vi "Sub_kalman_discrete_model.vi"() -> ()   [LabVIEW 2021]
uses:
  <vilib>/Analysis/Matrix/Datatypes/RealMatrix.ctl
  <vilib>/Analysis/7linalg.llb/Real Matrix Exp.vi
  <vilib>/Analysis/Matrix/Numeric/Multiply/Multiply - R,RM.vi
  <vilib>/Analysis/baseanly.llb/Real Inverse Matrix.vi
  <vilib>/Analysis/Matrix/Numeric/Subtract/Subtract - RM,RM.vi
  <vilib>/Analysis/Matrix/Numeric/Multiply/Multiply - RM,RM.vi
  <vilib>/Analysis/NI_AALBase.lvlib
  <vilib>/Analysis/Matrix/NI_Matrix.lvlib
panel:
  in  "control input?":bool
  out "A * B":T1
  out "H":T1
  in  "Sampling Time (s)":dbl format="%#.6p"
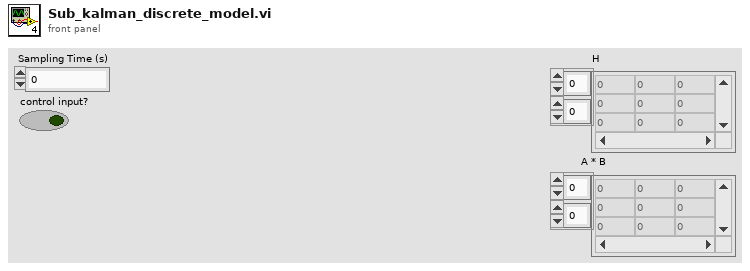
[diagram p1: front panel]
types:
  T1 = typedef "NI_Matrix.lvlib/RealMatrix.ctl" = dbl[][]
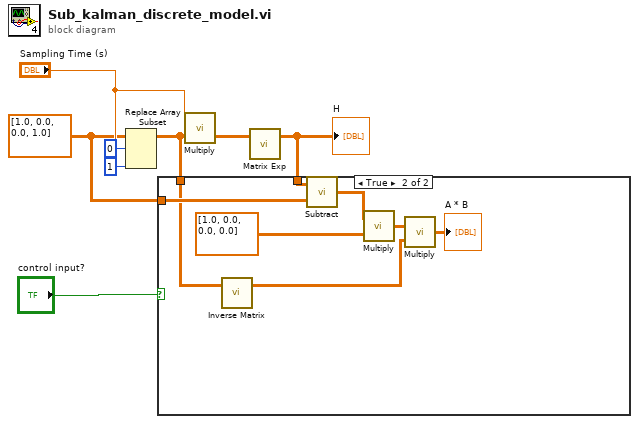
[diagram p0: block diagram]
diagram:
  w3 = T1 [[1.0, 0.0], [0.0, 1.0]] ("Matrix Exp")
  n1 = Replace Array Subset(array=w3, new element="Sampling Time (s)", index (row)=0, index (col)=1 ("disabled index (col)")) -> (w2:T1)
  n2 = call-poly <vilib>:"Multiply.vi"("Real Matrix A"=w2, "Real Scalar c"="Sampling Time (s)") -> ("c * A"=w6:T1)
  n3 = call-poly <vilib>:"Matrix Exp.vi"("Input Matrix"=w6) -> ("Matrix Exp"=w4:T1)  [unwired: 1 in, 1 out]
  "H" <- w4
  n4 = case shown="True" "control input?" {
    tunnel: w4 -> [_ w16]
    tunnel: w3 -> [_ w15]
    tunnel: w2 -> [_ w13]
    frame False {
    }
    frame True {
      n5 = call-poly <vilib>:"Inverse Matrix.vi"("Input Matrix"=w13) -> ("Inverse Matrix"=w11:T1)  [unwired: 1 in, 1 out]
      n6 = call-poly <vilib>:"Subtract.vi"("Real Matrix B"=w15, "Real Matrix A"=w16) -> ("A - B"=w14:T1)
      n7 = call-poly <vilib>:"Multiply.vi"("Real Matrix B"=T1 [[1.0, 0.0], [0.0, 0.0]] ("Matrix Exp"), "Real Matrix A"=w14) -> ("A * B"=w12:T1)
      n8 = call-poly <vilib>:"Multiply.vi"("Real Matrix B"=w11, "Real Matrix A"=w12) -> ("A * B"=→"A * B":T1)
    }
  }
